vi "TestString.vi"() -> ()   [LabVIEW 2018, in "RW_Protocols.lvlib"]
uses:
  RW_Protocols.lvlib
panel:
  out "F-format string":string
  in  "Numeric":dbl
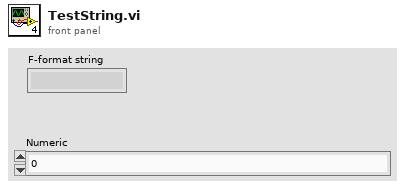
[diagram p1: front panel]
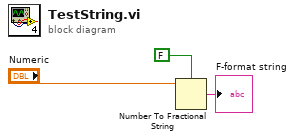
[diagram p0: block diagram]
diagram:
  n1 = Number To Fractional String(use system decimal point (T)=FALSE, number="Numeric") -> (F-format string=→"F-format string":string)  [unwired: 2 in]
